vi "ParaSet1.vi"(8 "Unit":bool, 9 "length":string, 10 "Speed":string, 11 "Mode":bool) -> (3 "String":string)   [LabVIEW 2014, in "Programing Logic.lvclass"]
uses:
  Programming Logic/Programing Logic.lvclass
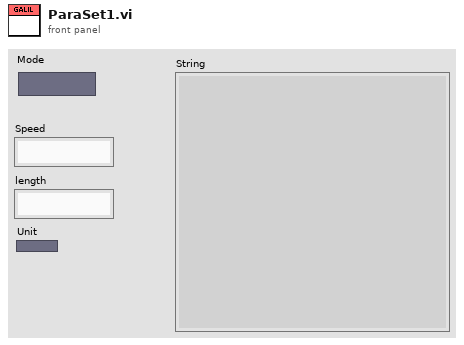
[diagram p1: front panel]
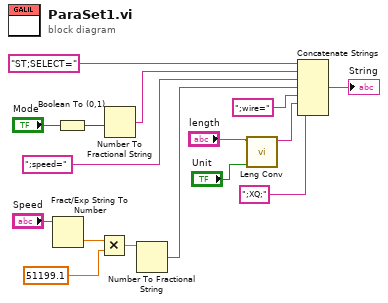
[diagram p0: block diagram]
diagram:
  n1 = Fract/Exp String To Number(string="Speed") -> (number=w11:dbl)  [unwired: 3 in, 1 out]
  n2 = Boolean To (0,1)(Boolean="Mode") -> (0, 1=w5:i16)
  n3 = Multiply(x=w11, y=51199.1) -> (x*y=w13:dbl)
  n4 = Number To Fractional String(number=w5) -> (F-format string=w4:string)  [unwired: 3 in]
  n5 = Number To Fractional String(number=w13) -> (F-format string=w14:string)  [unwired: 3 in]
  n6 = call "Leng Conv.vi"("Unit"="Unit", "length"="length") -> ("String"=w2:string)  [unwired: 9 in]
  n7 = Concatenate Strings("ST;SELECT=" ("string"), w4, ";speed=" ("string"), w14, ";wire=" ("string"), w2, ";XQ;" ("string")) -> (→"String":string)
